vi "Get Type.vi"(11 "Path 1D in":refnum<class "Path 1D.lvclass">) -> (3 "Type":string)   [LabVIEW 2020, in "Path 1D.lvclass"]
uses:
  <vilib>/gpm_packages/@cs/data-type-serializer/source/Path 1D/Path 1D.lvclass
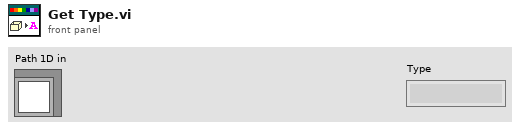
[diagram p1: front panel]
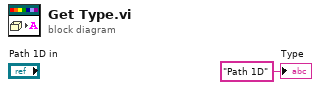
[diagram p0: block diagram]
diagram:
  "Type" <- "Path 1D" ("Type")
